vi "Obtain Request Events.vi"(8 "error in":errorcluster, 10 "Create New? (F)":bool) -> (0 "error out":errorcluster, 2 "SafetyLight Request Events":T1)   [LabVIEW 2025, in "SafetyLight.lvlib"]
doc: "This VI Obtains/Creates the Requests events that will be used for other modules to communicate with the module that owns this VI. These Requests events will be accessed only via Public API methods for this module.\n\n<b>NOTE</b>: The contents of this VI are automatically generated and modified by the <b>Tools > DQMH Consortium > DQMH</b> utilities. Consider using those utilities instead of making your own modifications to this VI.\n_____\nBased on DQMH Dev Tools: Project Template 7.1.0.1503."
uses:
  SafetyLight.lvlib
  Request Events--cluster.ctl
  Stop Argument--cluster.ctl
  Show Panel Argument--cluster.ctl
  Hide Panel Argument--cluster.ctl
  Get Module Execution Status Argument--cluster.ctl
  Show Diagram Argument--cluster.ctl
  Test Threshold Argument--cluster.ctl
  TestLight Argument--cluster.ctl
panel:
  # "NOTE: The contents of this VI are automatically generated and modified by the Tools > DQMH Consortium > DQMH utilities. Consider using those utilities instead of making your own modifications to this VI."
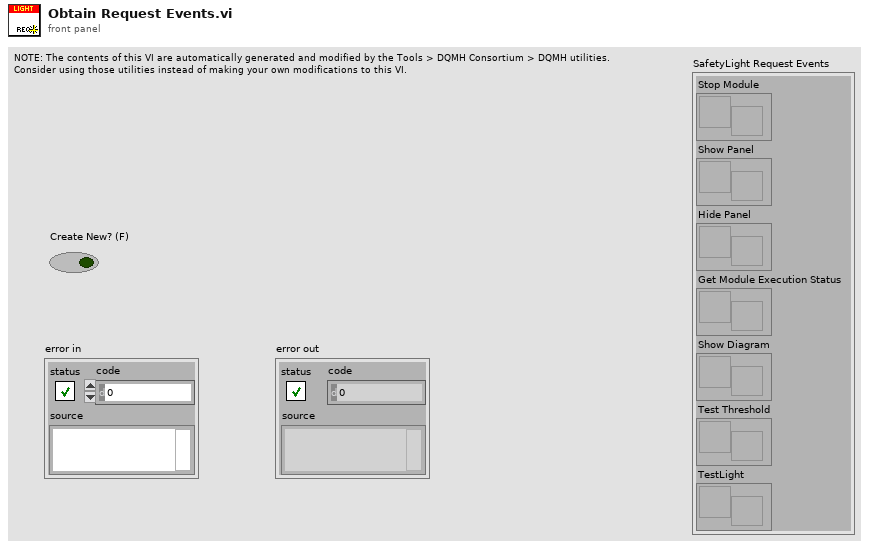
[diagram p1: front panel]
types:
  T1 = typedef "SafetyLight.lvlib/Request Events--cluster.ctl" = cluster{"Stop Module":refnum<user-event>, "Show Panel":refnum<user-event>, "Hide Panel":refnum<user-event>, "Get Module Execution Status":refnum<user-event>, "Show Diagram":refnum<user-event>, "Test Threshold":refnum<user-event>, "TestLight":refnum<user-event>}
  T2 = typedef "SafetyLight.lvlib/TestLight Argument--cluster.ctl" = cluster{"Desired State":bool}
  T3 = typedef "SafetyLight.lvlib/Test Threshold Argument--cluster.ctl" = cluster{"Numeric":dbl}
  T4 = typedef "SafetyLight.lvlib/Hide Panel Argument--cluster.ctl" = cluster{"Hide Panel?":bool}
  T5 = typedef "SafetyLight.lvlib/Show Panel Argument--cluster.ctl" = cluster{"Show Panel?":bool}
  T6 = typedef "SafetyLight.lvlib/Show Diagram Argument--cluster.ctl" = cluster{"Debug?":bool}
  T7 = typedef "SafetyLight.lvlib/Get Module Execution Status Argument--cluster.ctl" = cluster{"Running?":bool}
  T8 = typedef "SafetyLight.lvlib/Stop Argument--cluster.ctl" = cluster{"Origin":string, "Exit via Stop Module Req?":bool, "Wait for Module to stop?":bool}
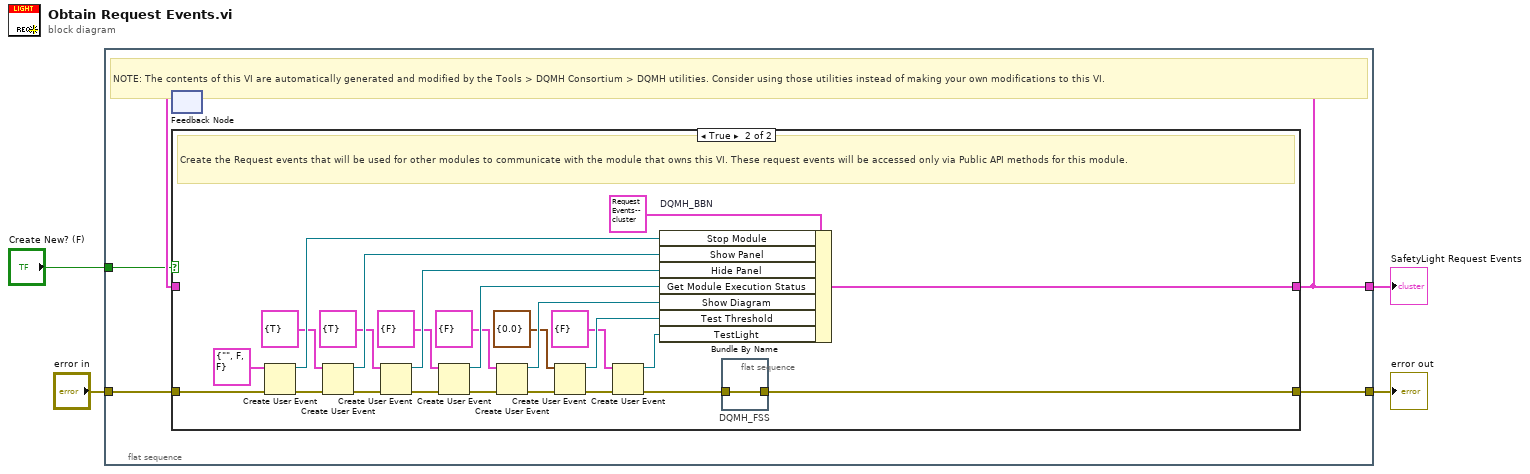
[diagram p0: block diagram]
diagram:
  n1 = flat-sequence {
    tunnel: [w9] -> w4
    tunnel: "error in" -> [w8]
    tunnel: [w6] -> w2
    tunnel: "Create New? (F)" -> [w5]
    frame #0 {
      # "NOTE: The contents of this VI are automatically generated and modified by the Tools > DQMH Consortium > DQMH utilities. Consider using those utilities instead of making your own modifications to this VI."
      n2 = feedback #1() -> (w7:T1)  [unwired: 1 in]
      n3 = case shown="True" w5 {
        tunnel: [w10 w26] -> w9
        tunnel: w8 -> [w10 w36]
        tunnel: [w11 w33] -> w6
        tunnel: w7 -> [w11 _]
        frame False {
          # "Obtain the Request events that were created in a previous call to this VI."
        }
        frame True {
          # "Create the Request events that will be used for other modules to communicate with the module that owns this VI. These request events will be accessed only via Public API methods for this module."
          n4 = Create User Event(user event datatype=T8 {"Origin"="", "Exit via Stop Module Req?"=FALSE, "Wait for Module to stop?"=FALSE} ("Stop Argument"), error in=w36) -> (user event=w34:refnum<user-event>, error out=w31:errorcluster)
          n5 = Create User Event(user event datatype=T5 {"Show Panel?"=TRUE} ("Show Panel Argument"), error in=w31) -> (user event=w30:refnum<user-event>, error out=w29:errorcluster)
          n6 = Create User Event(user event datatype=T4 {"Hide Panel?"=TRUE} ("Hide Panel Argument"), error in=w29) -> (user event=w28:refnum<user-event>, error out=w27:errorcluster)
          n7 = Create User Event(user event datatype=T7 {"Running?"=FALSE} ("Get Module Execution Status Argument"), error in=w27) -> (user event=w24:refnum<user-event>, error out=w25:errorcluster)
          n8 = Create User Event(user event datatype=T6 {"Debug?"=FALSE} ("Show Diagram Argument"), error in=w25) -> (user event=w21:refnum<user-event>, error out=w22:errorcluster)
          n9 = Create User Event(user event datatype=T3 {"Numeric"=0.0} ("Test Threshold Argument"), error in=w22) -> (user event=w16:refnum<user-event>, error out=w17:errorcluster)
          n10 = Create User Event(user event datatype=T2 {"Desired State"=FALSE} ("TestLight Argument"), error in=w17) -> (user event=w13:refnum<user-event>, error out=w14:errorcluster)
          n11 = Bundle By Name "DQMH_BBN"(cluster=T1 {"Stop Module"=refnum, "Show Panel"=refnum, "Hide Panel"=refnum, "Get Module Execution Status"=refnum, "Show Diagram"=refnum, "Test Threshold"=refnum, "TestLight"=refnum} ("output cluster"), "Stop Module"=w34, "Show Panel"=w30, "Hide Panel"=w28, "Get Module Execution Status"=w24, "Show Diagram"=w21, "Test Threshold"=w16, "TestLight"=w13) -> (w33:T1)
          n12 = flat-sequence "DQMH_FSS" {
            tunnel: w14 -> [w37]
            tunnel: [w37] -> w26
            frame #0 {
            }
          }
        }
      }
      n13 = feedback-in #1(w6) -> ()
    }
  }
  "SafetyLight Request Events" <- w2
  "error out" <- w4
